vi "Board Get Empty Space.vi"(8 "error in (no error)":errorcluster, 11 "Board in":refnum<class "Board.lvclass">) -> (0 "error out":errorcluster, 2 "Coordinate":T1, 3 "Board out":refnum<class "Board.lvclass">)   [LabVIEW 2019, in "Board.lvclass"]
uses:
  Board.lvclass
  <vilib>/numeric/Random Number (Range) U64.vi
  Coordinate STYP.ctl
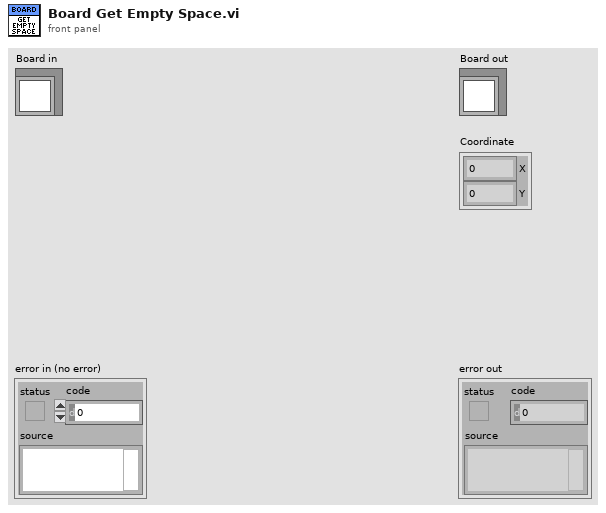
[diagram p1: front panel]
types:
  T1 = typedef "Coordinate STYP.ctl" = cluster{"X":i32, "Y":i32}
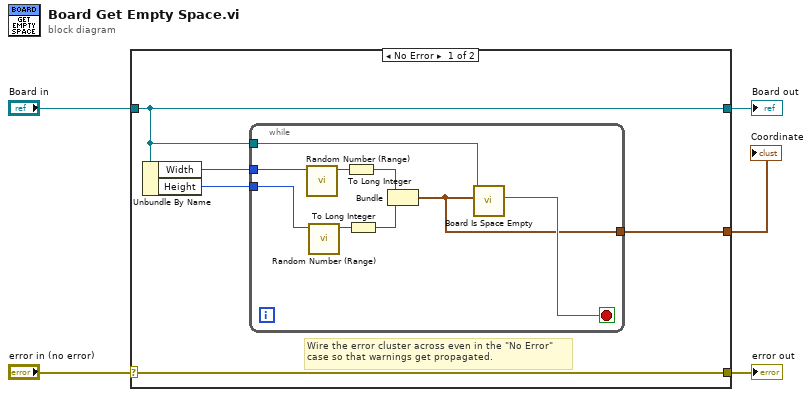
[diagram p0: block diagram]
diagram:
  n1 = case shown="No Error" "error in (no error)" {
    selector: "error in (no error)" -> [w10 w21]
    tunnel: [w10 w21] -> w4
    tunnel: [w9 w20] -> w2
    tunnel: "Board in" -> [w9 w20]
    tunnel: [w6 _] -> w1
    frame No Error {
      # "Wire the error cluster across even in the \"No Error\"\ncase so that warnings get propagated."
      n2 = Unbundle By Name(w9) -> ("Width"=w8:i32, "Height"=w7:i32)
      n3 = while {
        tunnel: w9 -> [w13]
        tunnel: w8 -> [w19]
        tunnel: w7 -> [w18]
        tunnel: [w11] -> w6
        stop <- w12 stop-if-true
        n4 = call-poly <vilib>:"Random Number (Range).vi"("upper bound (100)"=w19) -> ("number"=w17:u64)  [unwired: 10 in]
        n5 = call-poly <vilib>:"Random Number (Range).vi"("upper bound (100)"=w18) -> ("number"=w16:u64)  [unwired: 10 in]
        n6 = To Long Integer(number=w17) -> (32bit integer=w15:i32)
        n7 = To Long Integer(number=w16) -> (32bit integer=w14:i32)
        n8 = Bundle(w15, w14) -> (w11:cluster{i32, i32})  [unwired: 1 in]
        n9 = call-dynamic "Board Is Space Empty.vi"("Coordinate"=w11, "Board in"=w13) -> ("Empty?"=w12:bool)  [unwired: 7 in, 2 out]
      }
    }
    frame Error {
    }
  }
  "error out" <- w4
  "Board out" <- w2
  "Coordinate" <- w1
